vi "步进电机命令输入与输出1.vi"(2 "输入字符串":string, 3 "串口通信端口":refnum<visa-resource-name>) -> (0 "返回字符串":string, 1 "VISA资源名称输出":refnum<visa-resource-name>)   [LabVIEW 2016]
panel:
  # "步进电机命令输入与输出"
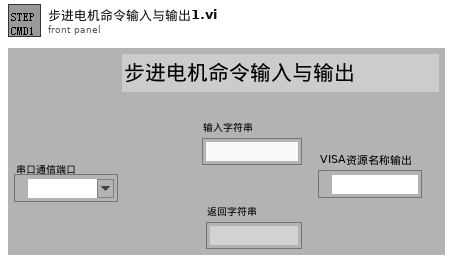
[diagram p1: front panel]
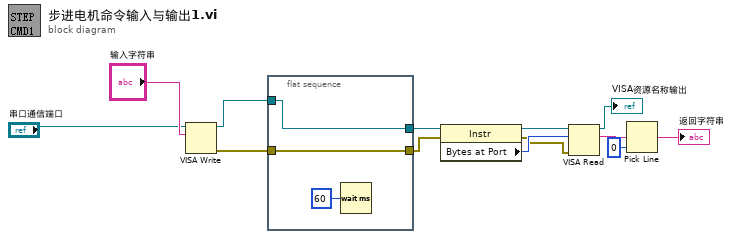
[diagram p0: block diagram]
diagram:
  n1 = VISA Write(VISA resource name="串口通信端口", write buffer="输入字符串") -> (VISA resource name out=w9:refnum<visa-resource-name>, error out=w8:errorcluster)  [unwired: 1 in, 1 out]
  n2 = flat-sequence {
    tunnel: w9 -> [w16]
    tunnel: w8 -> [w15]
    tunnel: [w16] -> w7
    tunnel: [w15] -> w6
    frame #0 {
      n3 = Wait (ms)(milliseconds to wait=u32 60 ("等待时间（毫秒）")) -> ()  [unwired: 1 out]
    }
  }
  n4 = property class="Instr"(reference=w7, error in=w6) -> (reference out=w11:refnum<visa-resource-name>, error out=w10:errorcluster, "Bytes at Port"=w12:u32)
  n5 = VISA Read(VISA resource name=w11, byte count=w12, error in (no error)=w10) -> (VISA resource name out=→"VISA资源名称输出":refnum<visa-resource-name>, read buffer=w4:string)  [unwired: 2 out]
  n6 = Pick Line(multi-line string=w4, line index=0 ("行索引")) -> (output string=→"返回字符串":string)  [unwired: 1 out]
